vi "BuildVectorplotScript.vi"(7 "datafilePath":path, 9 "PlotTitle":string="X = ") -> (3 "String out":string)   [LabVIEW 2013]
uses:
  minAndMax.ctl
  AutoManualNumber.ctl
  ticsAndGrids.ctl
  tics.ctl
  grids.ctl
  legendProperties.ctl
  legendAppearance.ctl
  alignment.ctl
  at.ctl
  axisName.ctl
panel:
  in  "Tab Control":enum32{"General", "Axes", "scriptOut"}(tab)
  in  "Height (in)":dbl=3.0 min=0.5 step=0.5 format="%.1f"
  in  "Width (in)":dbl=10.0 min=0.5 step=0.5 format="%.1f"
  in  "Set?":bool=TRUE
  in  "VectorScale":dbl=400.0
  in  "vectorLegendText":string
  in  "ShowLegend?":bool=TRUE
  in  "LegendProperties":T1={"Appearance"={"layout"="", "text-sample order"="", "key order"="", "surroundingBox"=""}, "Alignment"={"Horizontal"="", "Vertical"=""}, "Location"="auto", "\"At\" location"={"XcoordSys"="", "YcoordSys"="", "Xvalue"=0.0, "Yvalue"=0.0}}
  in  "xAxisBounds":T5={"Min"={"Auto"=TRUE, "Value"=0.0}, "Max"={"Auto"=TRUE, "Value"=0.0}}
  in  "yAxisBounds":T5={"Min"={"Auto"=TRUE, "Value"=0.0}, "Max"={"Auto"=TRUE, "Value"=0.0}}
  in  "X/Theta tics And Grids":T7={"tics"={"ticMin"=0.0, "ticStep"=0.0, "ticMax"=0.0, "minorDivsPerMajor"=2, "ticSpacing"=enum."Auto Tics", "ticPosition"=enum."Invisible"}, "Grids"={"Gridlines"=enum."No grids", "Zeroaxis"=enum."No zero axis"}, "Mapping"=enum."Lin"}
  in  "Y/R tics And Grids":T7={"tics"={"ticMin"=0.0, "ticStep"=0.0, "ticMax"=0.0, "minorDivsPerMajor"=2, "ticSpacing"=enum."Auto Tics", "ticPosition"=enum."Invisible"}, "Grids"={"Gridlines"=enum."No grids", "Zeroaxis"=enum."No zero axis"}, "Mapping"=enum."Lin"}
  in  "X Axis Label":string="Y(mm)"
  in  "Y Axis Label":string="Z(mm)"
  in  "AdditionalXTics":dbl[](array[numeric])
  in  "AdditionalYTics":dbl[](array[numeric])
  in  "ShowXLabel?":bool
  in  "ShowYLabel?":bool
  in  "ShowXNumbers?":bool
  in  "ShowYNumbers?":bool
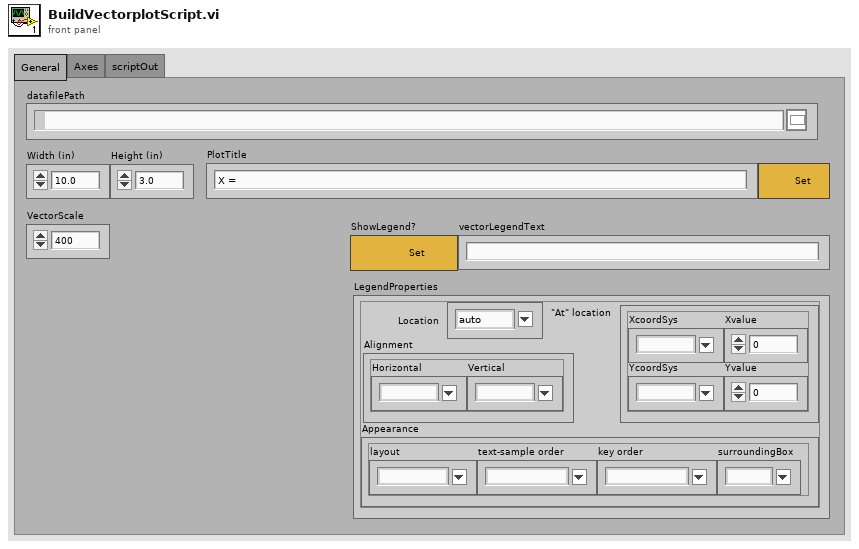
[diagram p1: front panel]
types:
  T1 = typedef "legendProperties.ctl" = cluster{"Appearance":T2, "Alignment":T3, "Location":string, "\"At\" location":T4}
  T2 = typedef "legendAppearance.ctl" = cluster{"layout":string, "text-sample order":string, "key order":string, "surroundingBox":string}
  T3 = typedef "alignment.ctl" = cluster{"Horizontal":string, "Vertical":string}
  T4 = typedef "at.ctl" = cluster{"XcoordSys":string, "YcoordSys":string, "Xvalue":dbl, "Yvalue":dbl}
  T5 = typedef "minAndMax.ctl" = cluster{"Min":T6, "Max":T6}
  T6 = typedef "AutoManualNumber.ctl" = cluster{"Auto":bool, "Value":dbl}
  T7 = typedef "ticsAndGrids.ctl" = cluster{"tics":T8, "Grids":T9, "Mapping":enum8{"Lin", "Log"}}
  T8 = typedef "tics.ctl" = cluster{"ticMin":dbl, "ticStep":dbl, "ticMax":dbl, "minorDivsPerMajor":i32, "ticSpacing":enum16{"Auto Tics", "Fixed spacing", "Fixed Minimum and Spacing", "Start, Spacing and Maximum", "Approx n Tics (rounded)"}, "ticPosition":enum16{"Inside, no mirror", "Inside, mirrored", "Outside, no mirror", "Outside, mirrored", "Invisible"}}
  T9 = typedef "grids.ctl" = cluster{"Gridlines":enum16{"No grids", "Major grid", "Minor grid", "Major and Minor"}, "Zeroaxis":enum16{"No zero axis", "Show zero axis"}}
  T10 = typedef "axisName.ctl" = string
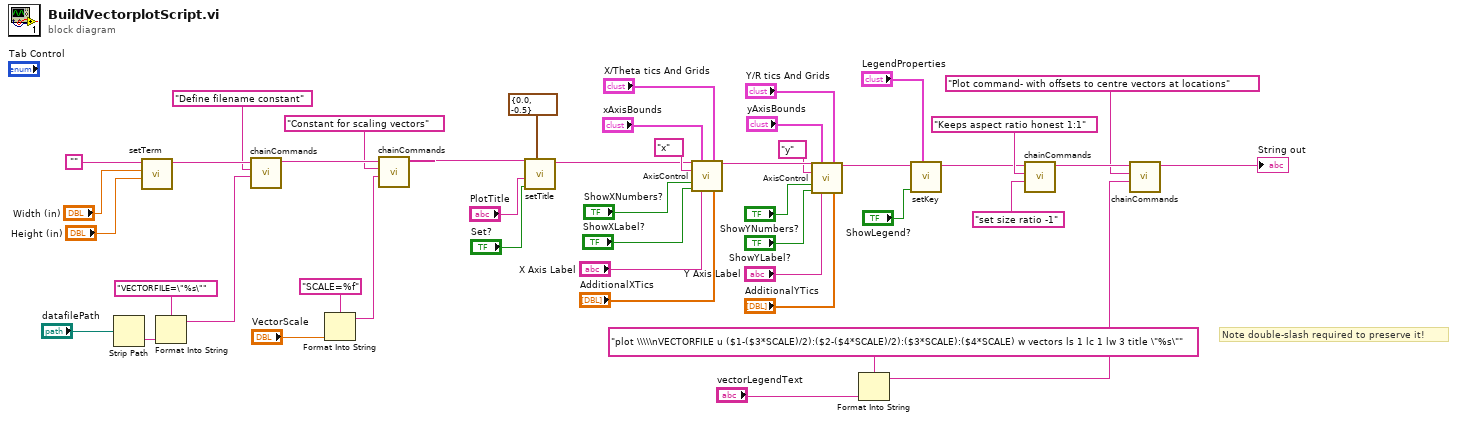
[diagram p0: block diagram]
diagram:
  # "Note double-slash required to preserve it!"
  n1 = Strip Path(path="datafilePath") -> (name=w22:string)  [unwired: 1 out]
  n2 = call "setTerm.vi"("Height (in)"="Height (in)", "Width (in)"="Width (in)", "String in"="") -> ("String out"=w20:string)  [unwired: 7 in, 1 out]
  n3 = Format Into String(format string="VECTORFILE=\"%s\"" ("string"), w22) -> (resulting string=w17:string)  [unwired: 2 in, 1 out]
  n4 = call "chainCommands.vi"("Command"=w17, "Comments"="Define filename constant", "StringIn"=w20) -> ("StringOut"=w19:string)  [unwired: 8 in]
  n5 = Format Into String(format string="SCALE=%f" ("string"), "VectorScale") -> (resulting string=w12:string)  [unwired: 2 in, 1 out]
  n6 = call "chainCommands.vi"("Command"=w12, "Comments"="Constant for scaling vectors", "StringIn"=w19) -> ("StringOut"=w18:string)  [unwired: 8 in]
  n7 = call "setTitle.vi"("Offset"=cluster{"horizontal":dbl, "vertical":dbl} {"horizontal"=0.0, "vertical"=-0.5}, "Set?"="Set?", "Title"="PlotTitle", "String in"=w18) -> ("String out"=w30:string)  [unwired: 6 in, 1 out]
  n8 = call "AxisControl.vi"("String in"=w30, "AxisBounds"="xAxisBounds", "ticsAndGrids"="X/Theta tics And Grids", "Axis"=T10 "x", "ShowNumbers?"="ShowXNumbers?", "ShowLabel?"="ShowXLabel?", "Axis Label"="X Axis Label", "AdditionalTics"="AdditionalXTics") -> ("String out"=w42:string)  [unwired: 6 in, 1 out]
  n9 = call "AxisControl.vi"("String in"=w42, "AxisBounds"="yAxisBounds", "ticsAndGrids"="Y/R tics And Grids", "Axis"=T10 "y", "ShowNumbers?"="ShowYNumbers?", "ShowLabel?"="ShowYLabel?", "Axis Label"="Y Axis Label", "AdditionalTics"="AdditionalYTics") -> ("String out"=w4:string)  [unwired: 6 in, 1 out]
  n10 = Format Into String(format string="plot \\\\\nVECTORFILE u ($1-($3*SCALE)/2):($2-($4*SCALE)/2):($3*SCALE):($4*SCALE) w vectors ls 1 lc 1 lw 3 title \"%s\"" ("string"), "vectorLegendText") -> (resulting string=w6:string)  [unwired: 2 in, 1 out]
  n11 = call "setKey.vi"("LegendProperties"="LegendProperties", "Set?"="ShowLegend?", "String in"=w4) -> ("String out"=w3:string)  [unwired: 7 in, 1 out]
  n12 = call "chainCommands.vi"("Command"="set size ratio -1", "Comments"="Keeps aspect ratio honest 1:1", "StringIn"=w3) -> ("StringOut"=w8:string)  [unwired: 8 in]
  n13 = call "chainCommands.vi"("Command"=w6, "Comments"="Plot command- with offsets to centre vectors at locations", "StringIn"=w8) -> ("StringOut"=→"String out":string)  [unwired: 8 in]
